vi "Master_Shutdown.vi"(8 "error in":errorcluster, 10 "FPGA VI Reference In":refnum<k20>) -> (0 "error out":errorcluster, 2 "FPGA VI Reference Out":refnum<k20>)   [LabVIEW 2018]
doc: "Disable all outputs and set all variables to a safe value before terminating connection with cRIO controller."
uses:
  CAN/TypeDef_BMSData.ctl
  CAN/TypeDef_BMS_Status.ctl
  Host/Libraries/TypeDef_CurrentState.ctl
  DAQ/Master_DataControl.ctl
  DAQ/TypeDef_cRIOData.ctl
  IMU/TypeDef_IMUData.ctl
  CAN/MotorController/fixedMotorData.ctl
  CAN/MotorController/MotorStatus.ctl
  <vilib>/Utility/error.llb/Error Cluster From Error Code.vi
  <vilib>/rvi/errors/niLvFpgaAdjustHostInterfaceError.vi
  <vilib>/rvi/interface/nirviReadWriteControl/nirviReadWriteControl.xnode
  <vilib>/NI_Real-Time Target Support.lvlib
  NiFpgaLv.dll
  <vilib>/rvi/interface/Simulation/niFpgaSimulationCallBeginRW.vi
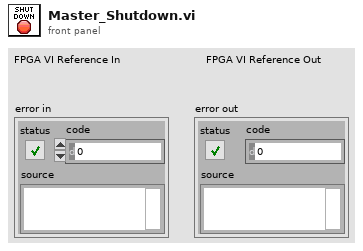
[diagram p1: front panel]
types:
  T1 = typedef "TypeDef_BMSData.ctl" = cluster{"Max Cell Voltage (V)":dbl, "Max Cell ID":dbl, "Min Cell Voltage (V)":dbl, "Min Cell ID":dbl, "State of Charge (%)":dbl, "Average Voltage (V)":dbl, "Voltage Delta (V)":dbl, "Pack Current (A)":dbl, "Pack Voltage (V)":dbl, "Max Resistance (Ohm)":dbl, "Min Resistance (Ohm)":dbl, "Average Resistance (Ohm)":dbl, "Delta Resistance (Ohm)":dbl, "Highest Temperature(F)":dbl, "BmsStatus":T2}
  T2 = typedef "TypeDef_BMS_Status.ctl" = cluster{"isFault":bool, "isolationMonitoring":bool}
  T3 = typedef "TypeDef_CurrentState.ctl" = enum16{"Fault", "Idle", "Ready", "Pushing", "Coast", "Braking"}
  T4 = typedef "Master_DataControl.ctl" = cluster{"cRIO Data":T5, "IMU Data":T6, "BMS Data":T1, "Motor Data":T7}
  T5 = typedef "TypeDef_cRIOData.ctl" = cluster{"Time (ms)":dbl, "24V Battery (V)":dbl, "LowV Current (A)":dbl, "Fiducial Sensor (V)":dbl, "PV Pressure (psig)":dbl, "Flow Sensor (V)":dbl, "Temp Fairing (F)":dbl, "Temp Reservoir (F)":dbl, "HallEffect Right (in)":dbl, "HallEffect Left (in)":dbl, "PT Tank (psig)":dbl, "PT Clamp Right (psig)":dbl, "PT Clamp Left (psig)":dbl, "PT Brake (psig)":dbl, "PT Cooling (psig)":dbl, "Displacement (ft)":dbl, "Velocity (ft/s)":dbl}
  T6 = typedef "TypeDef_IMUData.ctl" = cluster{"x acceleration (g)":dbl, "Pressure (psia)":dbl, "Temperature (F)":dbl}
  T7 = typedef "fixedMotorData.ctl" = cluster{"Velo (RPM)":dbl, "MotorTemp(F)":dbl, "CtrlTemp(F)":dbl, "DcLinkVolt(V)":dbl, "ErrorCode":dbl, "motorStatus":T8, "isAlive":bool, "motorControllerState":u16}
  T8 = typedef "MotorStatus.ctl" = cluster{"isReady":bool, "isOn":bool, "isOperEn":bool, "isFault":bool, "isVoltEn":bool, "targetReached":bool, "isWarning":bool}
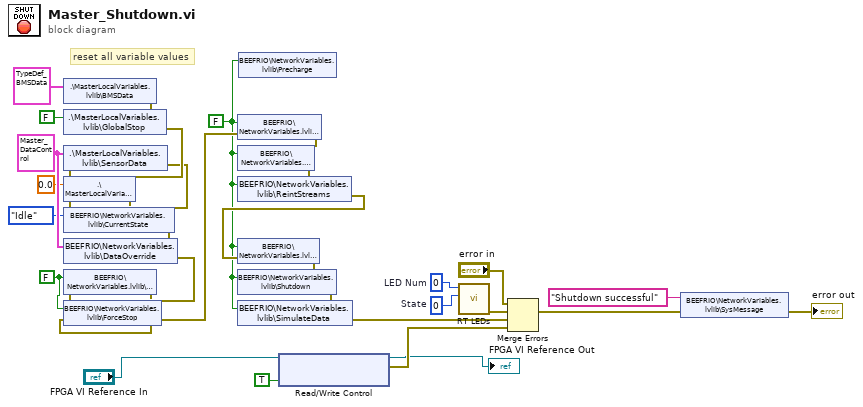
[diagram p0: block diagram]
diagram:
  w11 = FALSE ("ForceIdle")
  w14 = T4 {"cRIO Data"={"Time (ms)"=0.0, "24V Battery (V)"=0.0, "LowV Current (A)"=0.0, "Fiducial Sensor (V)"=0.0, "PV Pressure (psig)"=0.0, "Flow Sensor (V)"=0.0, "Temp Fairing (F)"=0.0, "Temp Reservoir (F)"=0.0, "HallEffect Right (in)"=0.0, "HallEffect Left (in)"=0.0, "PT Tank (psig)"=0.0, "PT Clamp Right (psig)"=0.0, "PT Clamp Left (psig)"=0.0, "PT Brake (psig)"=0.0, "PT Cooling (psig)"=0.0, "Displacement (ft)"=0.0, "Velocity (ft/s)"=0.0}, "IMU Data"={"x acceleration (g)"=0.0, "Pressure (psia)"=0.0, "Temperature (F)"=0.0}, "BMS Data"={"Max Cell Voltage (V)"=0.0, "Max Cell ID"=0.0, "Min Cell Voltage (V)"=0.0, "Min Cell ID"=0.0, "State of Charge (%)"=0.0, "Average Voltage (V)"=0.0, "Voltage Delta (V)"=0.0, "Pack Current (A)"=0.0, "Pack Voltage (V)"=0.0, "Max Resistance (Ohm)"=0.0, "Min Resistance (Ohm)"=0.0, "Average Resistance (Ohm)"=0.0, "Delta Resistance (Ohm)"=0.0, "Highest Temperature(F)"=0.0, "BmsStatus"={"isFault"=FALSE, "isolationMonitoring"=FALSE}}, "Motor Data"={"Velo (RPM)"=0.0, "MotorTemp(F)"=0.0, "CtrlTemp(F)"=0.0, "DcLinkVolt(V)"=0.0, "ErrorCode"=0.0, "motorStatus"={"isReady"=FALSE, "isOn"=FALSE, "isOperEn"=FALSE, "isFault"=FALSE, "isVoltEn"=FALSE, "targetReached"=FALSE, "isWarning"=FALSE}, "isAlive"=FALSE, "motorControllerState"=1}} ("SensorData")
  w3 = FALSE ("DumpValve")
  w31 = 0  # State
  w32 = 0  # LED Num
  # "reset all variable values"
  n1 = shared-variable ".\\MasterLocalVariables.lvlib\\BMSData"(T1 {"Max Cell Voltage (V)"=0.0, "Max Cell ID"=0.0, "Min Cell Voltage (V)"=0.0, "Min Cell ID"=0.0, "State of Charge (%)"=0.0, "Average Voltage (V)"=0.0, "Voltage Delta (V)"=0.0, "Pack Current (A)"=0.0, "Pack Voltage (V)"=0.0, "Max Resistance (Ohm)"=0.0, "Min Resistance (Ohm)"=0.0, "Average Resistance (Ohm)"=0.0, "Delta Resistance (Ohm)"=0.0, "Highest Temperature(F)"=0.0, "BmsStatus"={"isFault"=FALSE, "isolationMonitoring"=FALSE}} ("CANData")) -> (error out=w28:errorcluster)  [unwired: 1 in]
  n2 = shared-variable ".\\MasterLocalVariables.lvlib\\GlobalStop"(FALSE ("GlobalStop"), error in=w28) -> (error out=w27:errorcluster)
  n3 = shared-variable ".\\MasterLocalVariables.lvlib\\SensorData"(w14, error in=w27) -> (error out=w26:errorcluster)
  n4 = shared-variable ".\\MasterLocalVariables.lvlib\\Time"(0.0 ("Time"), error in=w26) -> (error out=w10:errorcluster)
  n5 = shared-variable "BEEFRIO\\NetworkVariables.lvlib\\CurrentState"(TypeDef_CurrentState."Idle" ("CurrentState"), error in=w10) -> (error out=w25:errorcluster)
  n6 = shared-variable "BEEFRIO\\NetworkVariables.lvlib\\DataOverride"(w14, error in=w25) -> (error out=w24:errorcluster)
  n7 = shared-variable "BEEFRIO\\NetworkVariables.lvlib\\ForceIdle"(w11, error in=w24) -> (error out=w23:errorcluster)
  n8 = shared-variable "BEEFRIO\\NetworkVariables.lvlib\\ForceStop"(w11, error in=w23) -> (error out=w17:errorcluster)
  n9 = shared-variable "BEEFRIO\\NetworkVariables.lvlib\\Launch"(w3, error in=w17) -> (error out=w22:errorcluster)
  n10 = shared-variable "BEEFRIO\\NetworkVariables.lvlib\\Ready"(w3, error in=w22) -> (error out=w21:errorcluster)
  n11 = shared-variable "BEEFRIO\\NetworkVariables.lvlib\\ReintStreams"(w3, error in=w21) -> (error out=w16:errorcluster)
  n12 = shared-variable "BEEFRIO\\NetworkVariables.lvlib\\Service"(w3, error in=w16) -> (error out=w20:errorcluster)
  n13 = shared-variable "BEEFRIO\\NetworkVariables.lvlib\\Shutdown"(w3, error in=w20) -> (error out=w19:errorcluster)
  n14 = shared-variable "BEEFRIO\\NetworkVariables.lvlib\\SimulateData"(w3, error in=w19) -> (error out=w18:errorcluster)
  n15 = shared-variable "BEEFRIO\\NetworkVariables.lvlib\\Precharge"(w3) -> ()  [unwired: 1 in, 1 out]
  n16 = xnode "Read/Write Control"("FPGA VI Reference In"="FPGA VI Reference In", "Pet RT Watchdog"=TRUE) -> ("FPGA VI Reference Out"=→"FPGA VI Reference Out":refnum<k20>, "error out"=w5:errorcluster)  [unwired: 1 in]
  n17 = call <vilib>:"RT LEDs.vi"("State"=w31, "LED Num"=w32) -> ("error out"=w29:errorcluster)  [unwired: 4 in, 1 out]
  n18 = Merge Errors("error in", w29, w18, w5) -> (w7:errorcluster)
  n19 = shared-variable "BEEFRIO\\NetworkVariables.lvlib\\SysMessage"("Shutdown successful" ("SysMessage"), error in=w7) -> (error out=→"error out":errorcluster)
